vi "getAndorErrorCodes.vi"(8 "error in (no error)":errorcluster, 11 "AndorIKonAcquisitor.lvclass in":refnum<class "AndorIKonAcquisitor.lvclass">) -> (0 "error out":errorcluster, 2 "Andor Error Codes":dbl[](array[numeric]), 3 "AndorIKonAcquisitor.lvclass out":refnum<class "AndorIKonAcquisitor.lvclass">)   [LabVIEW 2009, in "Hardware.lvlib" / "Channels.lvlib" / "AndorIKonAcquisitor.lvclass"]
uses:
  AndorIKonAcquisitor.lvclass
  AndorIKonAcquisitor.lvclass/AndorIKonAcquisitor.ctl
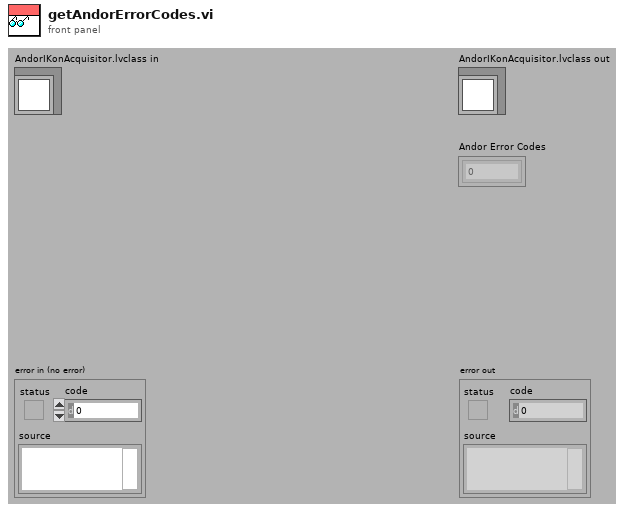
[diagram p1: front panel]
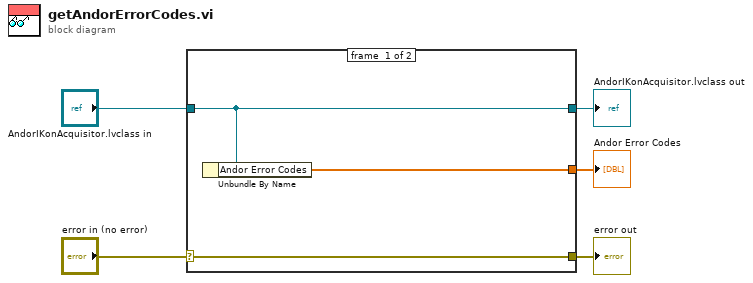
[diagram p0: block diagram]
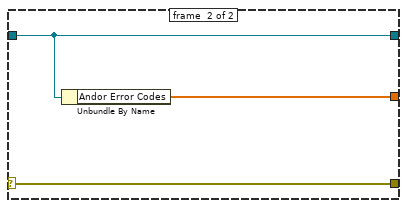
[diagram p2: hidden frame]
diagram:
  n1 = case shown="Error" "error in (no error)" {
    selector: "error in (no error)" -> [w8 w11]
    tunnel: [w8 w11] -> w4
    tunnel: [w7 w10] -> w2
    tunnel: "AndorIKonAcquisitor.lvclass in" -> [w7 w10]
    tunnel: [w6 w9] -> w1
    frame #0 {
      n2 = Unbundle By Name(w7) -> ("Andor Error Codes"=w6:dbl[])
    }
    frame #1 {
      n3 = Unbundle By Name(w10) -> ("Andor Error Codes"=w9:dbl[])
    }
  }
  "error out" <- w4
  "AndorIKonAcquisitor.lvclass out" <- w2
  "Andor Error Codes" <- w1
